vi "NormalizedIntensityVsRadius.vi"(8 "nBins":dbl, 9 "Min":dbl, 10 "Max":dbl, 11 "Input Array (r,I)":dbl[][](array[numeric])) -> (1 "Normalized Intensity":dbl[](array[numeric]), 2 "Radius bins":dbl[](array[numeric]), 3 "Normalized Intensity vs Radius":cluster{dbl[], dbl[]}(graph))   [LabVIEW 2016]
uses:
  <vilib>/Analysis/NI_AALPro.lvlib
panel:
  out "Histogram":i32[](array[numeric])
  out "Intensity Sum":dbl[](array[numeric])
  out "Bin width":dbl
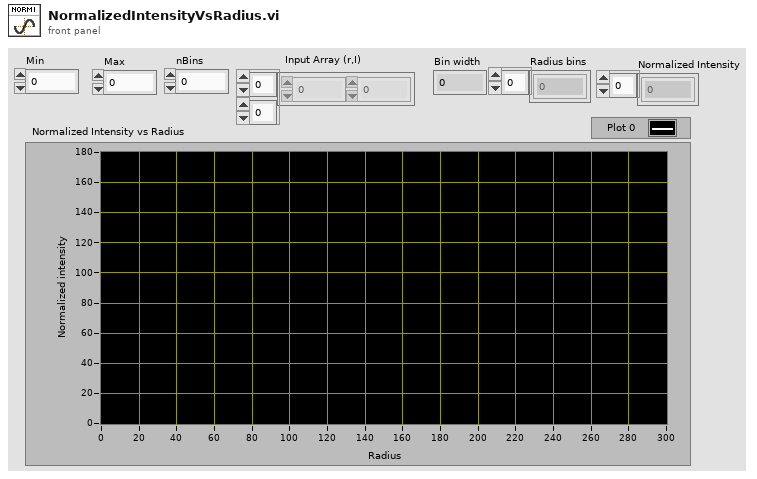
[diagram p1: front panel]
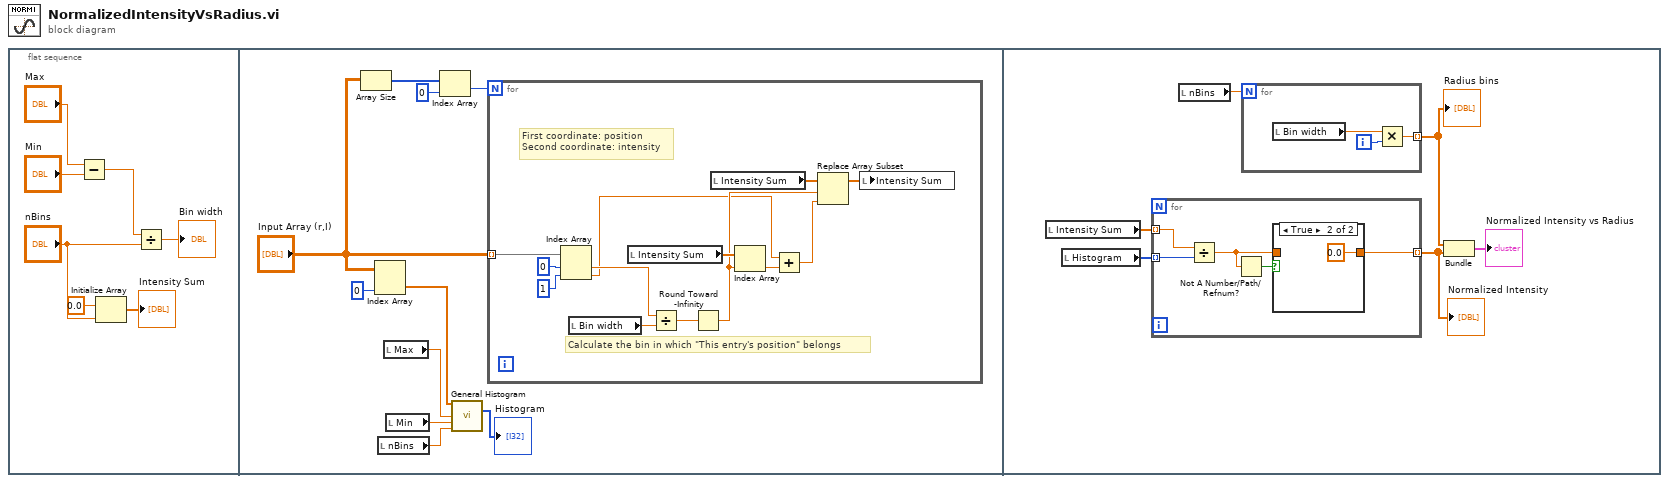
[diagram p0: block diagram]
diagram:
  n1 = flat-sequence {
    frame #0 {
      n2 = Subtract(x="Max", y="Min") -> (x-y=w4:dbl)
      n3 = Initialize Array(0.0 ("element"), "nBins") -> (→"Intensity Sum":dbl[])
      n4 = Divide(x=w4, y="nBins") -> (x/y=→"Bin width":dbl)
    }
    frame #1 {
      n5 = Array Size(array="Input Array (r,I)") -> (size(s)=w17:i32[])
      n6 = Index Array(array="Input Array (r,I)", index (col)=0 ("index")) -> (element=w12:dbl[])  [unwired: 1 in]
      n7 = local read "nBins"() -> (w9:dbl)
      n8 = local read "Max"() -> (w11:dbl)
      n9 = local read "Min"() -> (w10:dbl)
      n10 = Index Array(array=w17, index=0) -> (element=w15:i32)
      n11 = call <vilib>:"General Histogram.vi"("X"=w12, "max"=w11, "min"=w10, "# bins"=w9) -> ("Histogram"=→"Histogram":i32[])  [unwired: 7 in, 4 out]
      n12 = for {
        N: w15 -> [_]
        tunnel: "Input Array (r,I)" -> [w30] mode=indexing
        # "Calculate the bin in which \"This entry's position\" belongs"
        # "First coordinate: position\nSecond coordinate: intensity"
        n13 = Index Array(array=w30, index #1=0 ("index"), index #2=1 ("index")) -> (element #1=w19:dbl, element #2=w18:dbl)
        n14 = local read "Bin width"() -> (w27:dbl)
        n15 = local read "Intensity Sum"() -> (w25:dbl[])
        n16 = Divide(x=w19, y=w27) -> (x/y=w26:dbl)
        n17 = Round Toward -Infinity(1:w26) -> (0:w20:dbl)
        n18 = local read "Intensity Sum"() -> (w23:dbl[])
        n19 = Index Array(array=w25, index=w20) -> (element=w21:dbl)
        n20 = Add(x=w18, y=w21) -> (x+y=w24:dbl)
        n21 = Replace Array Subset(array=w23, new element=w24, index=w20) -> (w22:dbl[])
        n22 = local write "Intensity Sum"(w22) -> ()
      }
    }
    frame #2 {
      n23 = local read "Intensity Sum"() -> (w36:dbl[])
      n24 = local read "Histogram"() -> (w35:i32[])
      n25 = for {
        tunnel: w36 -> [w44] mode=indexing
        tunnel: w35 -> [w43] mode=indexing
        tunnel: [w40] -> w33 mode=indexing
        n26 = Divide(x=w44, y=w43) -> (x/y=w41:dbl)
        n27 = Not A Number/Path/Refnum?(number/path/refnum=w41) -> (NaN/Path/Refnum?=w42:bool)
        n28 = case shown="True" w42 {
          tunnel: [w45 0.0] -> w40
          tunnel: w41 -> [w45 _]
          frame False {
          }
          frame True {
          }
        }
      }
      "Normalized Intensity" <- w33
      n29 = local read "nBins"() -> (w32:dbl)
      n30 = for {
        N: w32 -> [_]
        tunnel: [w37] -> w31 mode=indexing
        i -> [w38]
        n31 = local read "Bin width"() -> (w39:dbl)
        n32 = Multiply(x=w39, y=w38) -> (x*y=w37:dbl)
      }
      "Radius bins" <- w31
      n33 = Bundle(w31, w33) -> (→"Normalized Intensity vs Radius":cluster{dbl[], dbl[]})  [unwired: 1 in]
    }
  }
